vi "LossyEnqueueMessage.vi"(8 "error in":errorcluster, 10 "Message":refnum<class "Message.lvclass">, 11 "MessageQueue in":refnum<class "MessageQueue.lvclass">) -> (0 "error out":errorcluster, 1 "Overflow?":bool, 2 "Overflow Message":refnum<class "Message.lvclass">, 3 "MessageQueue out":refnum<class "MessageQueue.lvclass">)   [LabVIEW 2017, in "LapDog.Messaging.v3.lvlib" / "MessageQueue.lvclass"]
doc: "Adds an element to the queue. If the queue is full, the first element is removed from the queue and returned to the caller.\n\nThis method executes regardless of the error in state."
uses:
  MessageQueue.lvclass
  Message/Message.lvclass
  MessageQueue.lvclass/MessageQueue.ctl
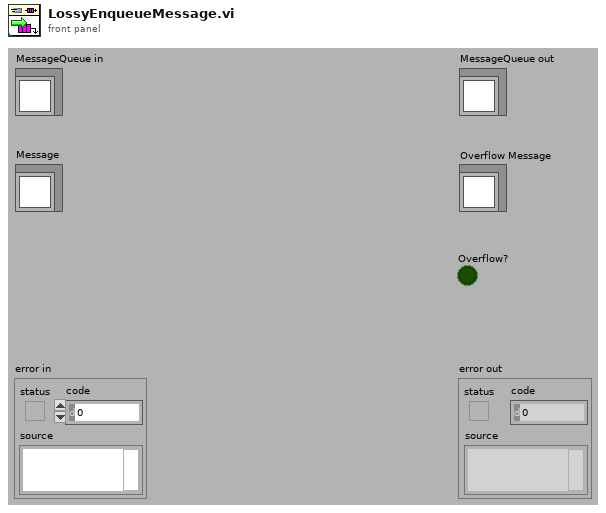
[diagram p1: front panel]
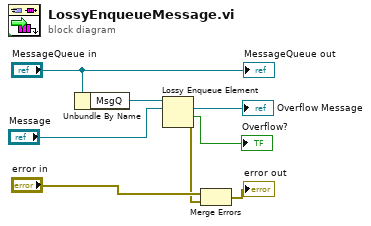
[diagram p0: block diagram]
diagram:
  n1 = Unbundle By Name("MessageQueue in") -> ("MsgQ"=w8:refnum<queue>)
  n2 = Lossy Enqueue Element(queue=w8, element="Message") -> (overflow element=→"Overflow Message":refnum<class "Message.lvclass">, overflow?=→"Overflow?":bool, error out=w1:errorcluster)  [unwired: 1 in, 1 out]
  n3 = Merge Errors("error in", w1) -> (→"error out":errorcluster)
  "MessageQueue out" <- "MessageQueue in"
